vi "SearchString.vi"(0 "String":string, 7 "Search string":string, 11 "Offset":i32 caption="Offset (0)") -> (4 "Substring before match":string, 8 "Rest of string":string, 15 "Offset past match":i32)   [LabVIEW 2017, in "GPString.lvlib"]
doc: "Searches for <B>Search string</B> in <B>String</B> starting from <B>Offset</B>.\n\nIf this function finds the search string <B>Substring before match</B>, <B>Rest of string</B>, and <B>Offset past match</B> will be returned.\n\nIf this function does not find the search string <B>Substring before match</B> will contain the entire <B>String</B>, <B>Rest of string</B> will be empty, and <B>Offset past match</B> will be -1.\n\nThis VI searches for an ordinary string like the built-in Search/Split String function does, but it strips away the search string itself like the built-in Match Pattern function. It is much faster than the Match Pattern function though, as this VI does not support regular expressions.\n\nThis VI is inlined.\n\nSteen Schmidt\nGPower\n13/11 2013"
uses:
  GPString.lvlib
panel:
  # "Copyright © 2016\nGPower\nSee enclosed license file for terms and conditions"
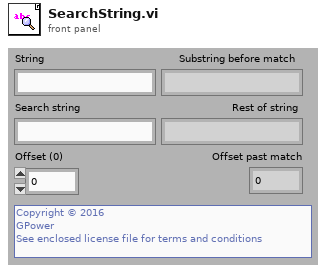
[diagram p1: front panel]
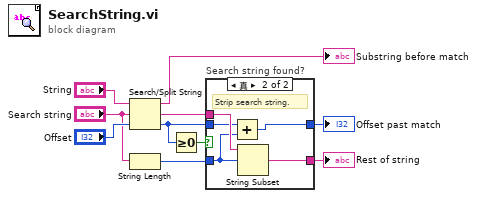
[diagram p0: block diagram]
diagram:
  n1 = Search/Split String(string="String", search string/char (-)="Search string", offset (0)="Offset") -> (substring before match=→"Substring before match":string, match + rest of string=w8:string, offset of match=w4:i32)
  n2 = String Length(string="Search string") -> (length=w6:i32)
  n3 = Greater Or Equal To 0?(x=w4) -> (x >= 0?=w5:bool)
  n4 = case "Search string found?" shown="真" w5 {
    tunnel: w8 -> [_ w16]
    tunnel: w6 -> [_ w14]
    tunnel: w4 -> [w11 w15]
    tunnel: [w11 w13] -> w2
    tunnel: [_ w12] -> w1
    frame False {
    }
    frame True {
      # "Strip search string."
      n5 = Add(x=w15, y=w14) -> (x+y=w13:i32)
      n6 = String Subset(string=w16, offset (0)=w14) -> (substring=w12:string)  [unwired: 1 in]
    }
  }
  "Rest of string" <- w1
  "Offset past match" <- w2
